vi "Queue Add Events to Front.vi"(7 "State Array":cluster{"State":string}[](array[cluster]), 8 "Error In":errorcluster, 11 "Queue In":refnum<queue>) -> (0 "Error Out":errorcluster, 3 "Queue Out":refnum<queue>)   [LabVIEW 2015]
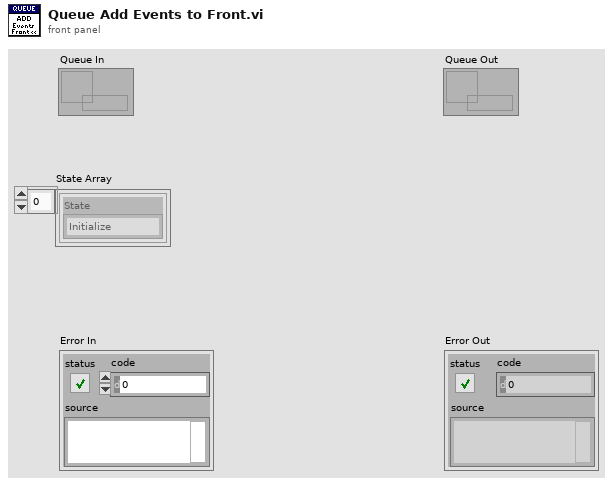
[diagram p1: front panel]
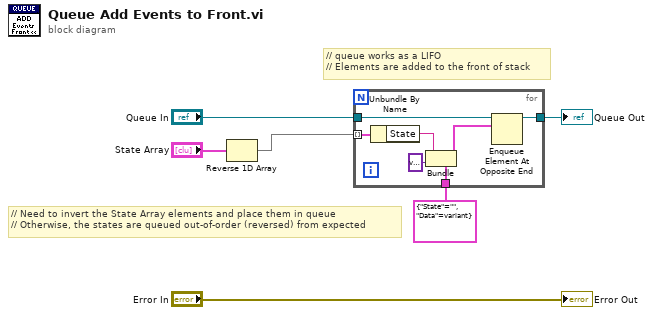
[diagram p0: block diagram]
diagram:
  # "// Need to invert the State Array elements and place them in queue\n// Otherwise, the states are queued out-of-order (reversed) from expected"
  # "// queue works as a LIFO\n// Elements are added to the front of stack"
  n1 = Reverse 1D Array(array="State Array") -> (reversed array=w1:cluster{"State":string}[])
  n2 = for {
    tunnel: w1 -> [w10] mode=indexing
    tunnel: "Queue In" -> [w13]
    tunnel: [w12] -> w3
    tunnel: cluster{"State":string, "Data":variant} {"State"="", "Data"=variant} ("Cluster") -> [w11]
    n3 = Unbundle By Name(w10) -> ("State"=w9:string)
    n4 = Bundle(cluster=w11, "State"=w9, "Data"=variant) -> (w7:cluster{"State":string, "Data":variant})
    n5 = Enqueue Element At Opposite End(queue=w13, element=w7) -> (queue out=w12:refnum<queue>)  [unwired: 2 in, 2 out]
  }
  "Queue Out" <- w3
  "Error Out" <- "Error In"
